vi "LibXML_GetAllAttributes.vi"(8 "error in":errorcluster, 9 "attr. name":string="/ScanMaster/Devices/Device/description", 10 "xpathexpr (root)":string="/ScanMaster/Devices/Device/description", 11 "doc":u32) -> (0 "error out":errorcluster, 1 "value list":string[](array[string]), 2 "value":string="the piezo x axis via adwin analog out", 3 "doc copy out":u32, 4 "#ofNodes":u32)   [LabVIEW 2019, in "Tools.lvlib" / "LibXML.lvlib"]
doc: "Get all attributes at XPath with attribute name in doc."
uses:
  LibXML.lvlib
  Error Cluster From Error Code_subroutine.vi
  <vilib>/Utility/error.llb/Trim Whitespace.vi
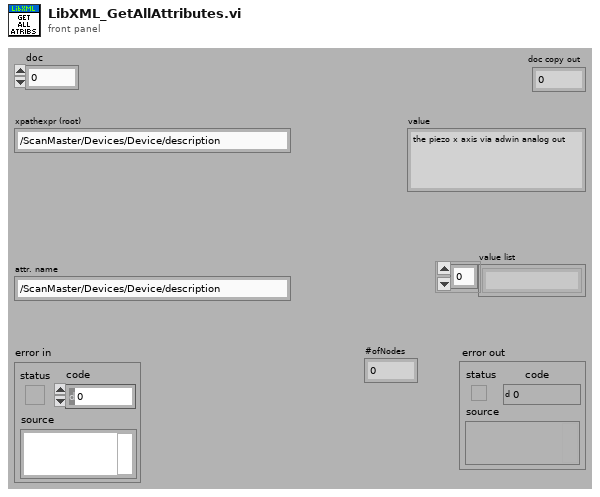
[diagram p1: front panel]
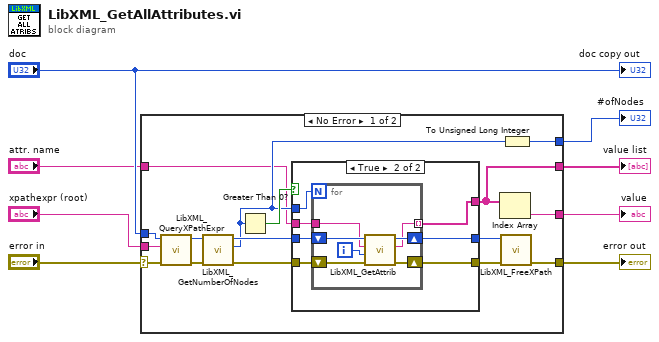
[diagram p0: block diagram]
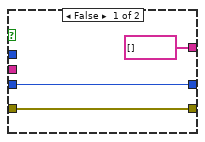
[diagram p2: hidden frame]
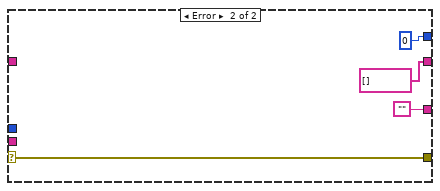
[diagram p3: hidden frame]
diagram:
  n1 = case shown="No Error" "error in" {
    selector: "error in" -> [w10 w43]
    tunnel: "xpathexpr (root)" -> [w22 _]
    tunnel: [w20 ""] -> w7
    tunnel: "doc" -> [w18 _]
    tunnel: [w16 string[] []] -> w5
    tunnel: [w9 u32 0] -> w4
    tunnel: [w13 w43] -> w3
    tunnel: "attr. name" -> [w11 _]
    frame No Error {
      n2 = call "LibXML_QueryXPathExpr.vi"("error in"=w10, "XPathExpr"=w22, "doc"=w18) -> ("error out"=w24:errorcluster, "xmlXPathObj"=w21:u32)  [unwired: 7 in]
      n3 = call "LibXML_GetNumberOfNodes.vi"("error in (no error)"=w24, "XPathObj"=w21) -> ("error out"=w23:errorcluster, "#ofNodes"=w15:i32, "XPathObj out"=w19:u32)  [unwired: 7 in]
      n4 = Greater Than 0?(x=w15) -> (x > 0?=w17:bool)
      n5 = case shown="True" w17 {
        tunnel: w23 -> [w27 w34]
        tunnel: w19 -> [w25 w33]
        tunnel: [w27 w32] -> w12
        tunnel: [string[] [] w31] -> w16
        tunnel: w15 -> [_ w30]
        tunnel: [w25 w29] -> w14
        tunnel: w11 -> [_ w28]
        frame False {
        }
        frame True {
          n6 = for {
            N: w30 -> [_]
            shift-right: [w40] -> w32
            shift-left: w34 -> [w41]
            shift-right: [w37] -> w29
            shift-left: w33 -> [w38]
            tunnel: [w36] -> w31 mode=indexing
            tunnel: w28 -> [w35]
            i -> [w39]
            n7 = call "LibXML_GetAttrib.vi"("error in"=w41, "index"=w39, "attribute"=w35, "XPathObj"=w38) -> ("error out"=w40:errorcluster, "value"=w36:string, "XPathObj out"=w37:u32)  [unwired: 4 in, 1 out]
          }
        }
      }
      n8 = Index Array(array=w16) -> (element=w20:string)  [unwired: 1 in]
      n9 = call "LibXML_FreeXPath.vi"("error in"=w12, "XPathObj"=w14) -> ("error out"=w13:errorcluster)  [unwired: 9 in]
      n10 = To Unsigned Long Integer(number=w15) -> (unsigned 32bit integer=w9:u32)
    }
    frame Error {
    }
  }
  "value" <- w7
  "#ofNodes" <- w4
  "error out" <- w3
  "value list" <- w5
  "doc copy out" <- "doc"
